vi "Initialize.vi"(8 "error in (no error)":errorcluster, 11 "Component Settings Editor in":refnum<class "Component Settings Editor.lvclass">) -> (0 "error out":errorcluster, 3 "Component Settings Editor out":refnum<class "Component Settings Editor.lvclass">)   [LabVIEW 2020, in "DSF Core.lvlib" / "Component Settings Editor.lvclass"]
uses:
  Component Settings Editor.lvclass
  Component Settings Editor.lvclass/Component Settings Editor.ctl
  User Interface.lvclass
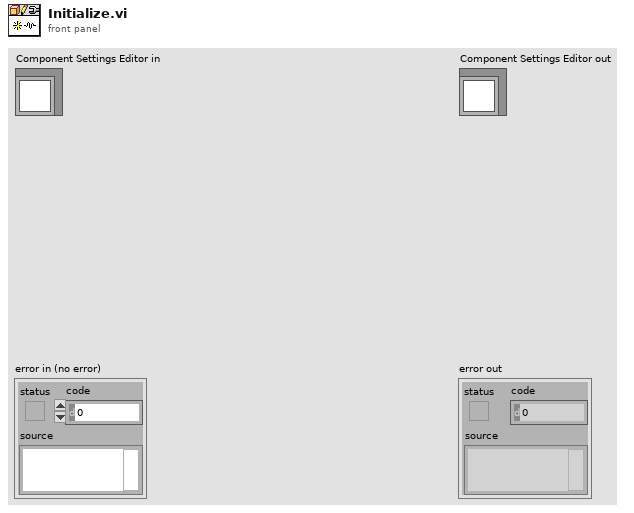
[diagram p1: front panel]
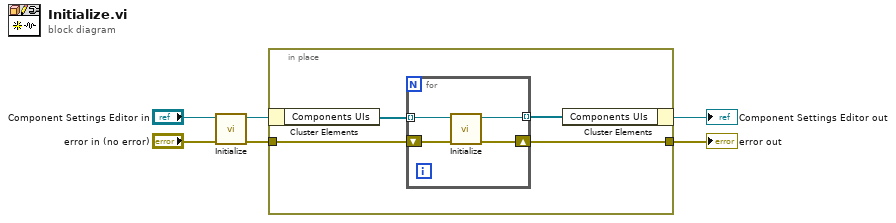
[diagram p0: block diagram]
diagram:
  n1 = call-parent "Initialize.vi"("error in (no error)"="error in (no error)", "User Interface in"="Component Settings Editor in") -> ("error out"=w4:errorcluster, "User Interface out"=w3:refnum<class "Component Settings Editor.lvclass">)  [unwired: 8 in]
  n2 = in-place {
    in-place-border: w4 -> [w10]
    in-place-border: [w7] -> w2
    n3 = in-place-cluster #1(w3) -> ("Components UIs"=w9:refnum<class "User Interface.lvclass">[])
    n4 = for {
      tunnel: w9 -> [w13] mode=indexing
      shift-right: [w12] -> w7
      shift-left: w10 -> [w14]
      tunnel: [w11] -> w8 mode=indexing
      n5 = call-dynamic "Initialize.vi"("error in (no error)"=w14, "User Interface in"=w13) -> ("error out"=w12:errorcluster, "User Interface out"=w11:refnum<class "User Interface.lvclass">)  [unwired: 8 in]
    }
    n6 = in-place-cluster #1("Components UIs"=w8) -> (→"Component Settings Editor out":refnum<class "Component Settings Editor.lvclass">)
  }
  "error out" <- w2
